vi "ConfigureRegulators.vi"(0 "axis in":cluster{"keyHandle":u32, "nodeId":u16}={"keyHandle"=0, "nodeId"=1}, 5 "position gains":T1, 7 "velocity gains":cluster{"p-Gain":u16, "i-Gain":u16}, 9 "current gains":cluster{"p-Gain":u16, "i-Gain":u16}, 11 "error in (no error)":errorcluster) -> (4 "axis out":cluster{"keyHandle":u32, "nodeId":u16}={"keyHandle"=0, "nodeId"=1}, 15 "error out":errorcluster)   [LabVIEW 2018]
doc: "<B>ConfigureRegulators</B> writes the regulation gain parameters to the device."
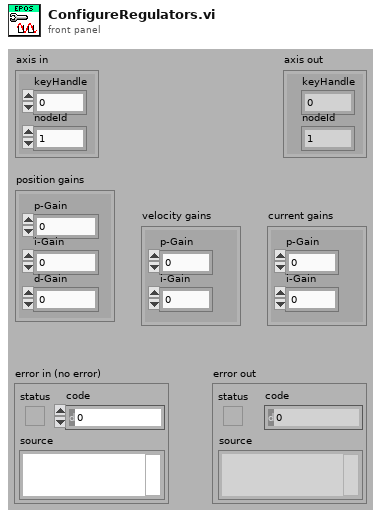
[diagram p1: front panel]
types:
  T1 = cluster{"p-Gain":u16, "i-Gain":u16, "d-Gain":u16}
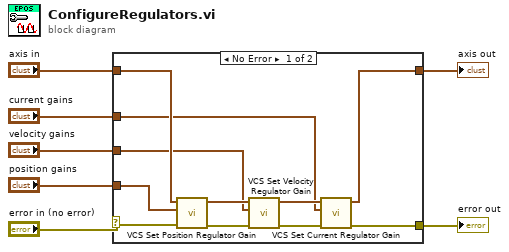
[diagram p0: block diagram]
diagram:
  n1 = case shown="No Error" "error in (no error)" {
    selector: "error in (no error)" -> [w18 w20]
    tunnel: [w15 w20] -> w6
    tunnel: [w14 w19] -> w5
    tunnel: "axis in" -> [w11 w19]
    tunnel: "position gains" -> [w10 _]
    tunnel: "velocity gains" -> [w9 _]
    tunnel: "current gains" -> [w8 _]
    frame No Error {
      n2 = call "VCS Set Position Regulator Gain.vi"("error in (no error)"=w18, "gains"=w10, "axis in"=w11) -> ("error out"=w17:errorcluster, "axis out"=w12:cluster{"keyHandle":u32, "nodeId":u16})  [unwired: 7 in]
      n3 = call "VCS Set Velocity Regulator Gain.vi"("error in (no error)"=w17, "gains"=w9, "axis in"=w12) -> ("error out"=w16:errorcluster, "axis out"=w13:cluster{"keyHandle":u32, "nodeId":u16})  [unwired: 7 in]
      n4 = call "VCS Set Current Regulator Gain.vi"("error in (no error)"=w16, "gains"=w8, "axis in"=w13) -> ("error out"=w15:errorcluster, "axis out"=w14:cluster{"keyHandle":u32, "nodeId":u16})  [unwired: 7 in]
    }
    frame Error {
    }
  }
  "error out" <- w6
  "axis out" <- w5
